vi "Write Modified.vi"(8 "error in (no error)":errorcluster, 10 "Modified?":bool, 11 "LabVIEW-Config In":refnum<class "LabVIEW-Config.lvclass">) -> (0 "error out":errorcluster, 3 "LabVIEW-Config Out":refnum<class "LabVIEW-Config.lvclass">)   [LabVIEW 2017, in "LabVIEW-Config.lvlib" / "LabVIEW-Config.lvclass"]
uses:
  LabVIEW-Config.lvclass
  LabVIEW-Config.lvclass/LabVIEW-Config.ctl
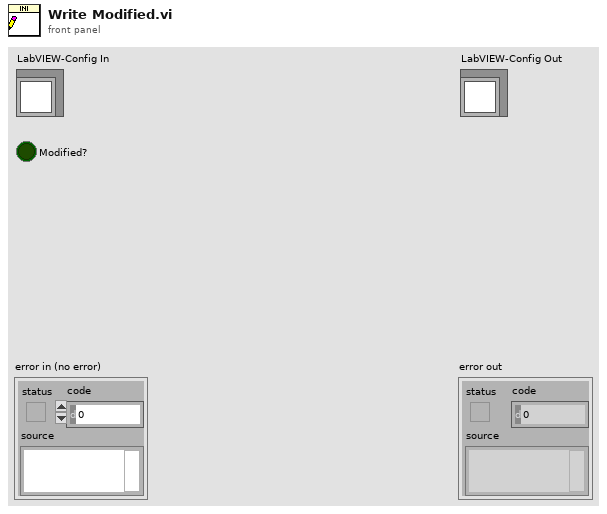
[diagram p1: front panel]
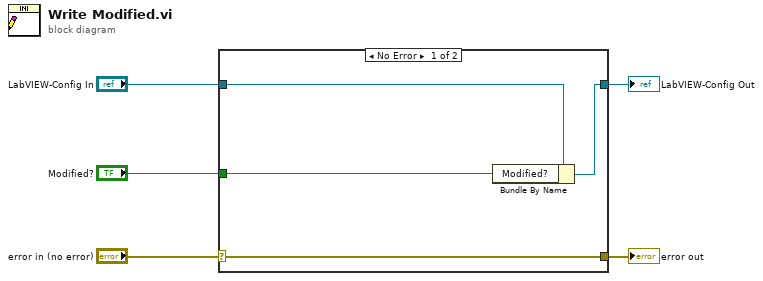
[diagram p0: block diagram]
diagram:
  n1 = case shown="No Error" "error in (no error)" {
    selector: "error in (no error)" -> [w9 w10]
    tunnel: [w9 w10] -> w4
    tunnel: [w7 w11] -> w2
    tunnel: "LabVIEW-Config In" -> [w8 w11]
    tunnel: "Modified?" -> [w6 _]
    frame No Error {
      n2 = Bundle By Name(cluster=w8, "Modified?"=w6) -> (w7:refnum<class "LabVIEW-Config.lvclass">)
    }
    frame Error {
    }
  }
  "error out" <- w4
  "LabVIEW-Config Out" <- w2
